vi "ASCII转字符串.vi"() -> ()   [LabVIEW 2013]
panel:
  out "数值":dbl
  out "字符串 3":string
  in  "字符串 2":string
  in  "字符串":string
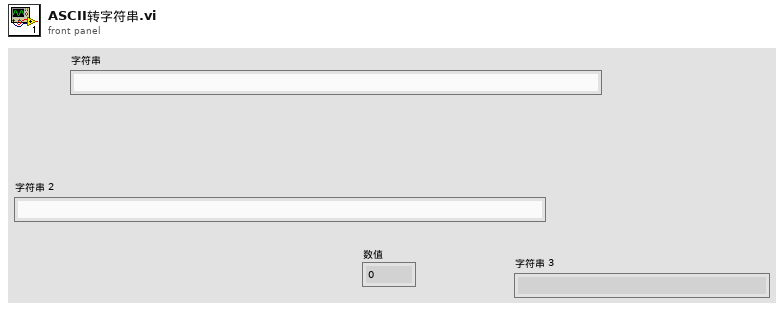
[diagram p1: front panel]
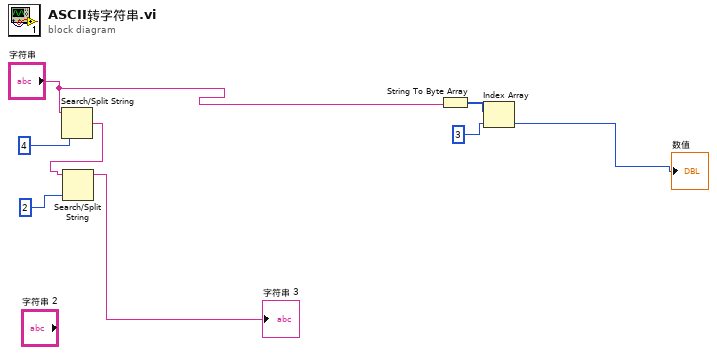
[diagram p0: block diagram]
diagram:
  n1 = Search/Split String(string="字符串", offset (0)=4) -> (match + rest of string=w6:string)  [unwired: 1 in, 2 out]
  n2 = Search/Split String(string=w6, offset (0)=2) -> (substring before match=→"字符串 3":string)  [unwired: 1 in, 2 out]
  n3 = String To Byte Array(string="字符串") -> (unsigned byte array=w5:u8[])
  n4 = Index Array(array=w5, index=3) -> (element=→"数值":u8)
